vi "Log (single).vi"(8 "error in (no error)":errorcluster, 10 "Type":enum16{"Ln", "Log"}(ring), 11 "XY-data":cluster{"X-array":dbl[], "Y-array":dbl[]} {"Y-array" format="%.2p"; "X-array" format="%.2p"}) -> (0 "error out":errorcluster, 3 "XY-data out":cluster{"X-array":dbl[], "Y-array":dbl[]} {"Y-array" format="%.2p"; "X-array" format="%.2p"})   [LabVIEW 2019, in "xy_utilities.lvlib"]
doc: "Square <b>XY-data</b>'s y array.\n\nWire data to the data input to determine the polymorphic instance to use or manually select the instance."
uses:
  xy_utilities.lvlib
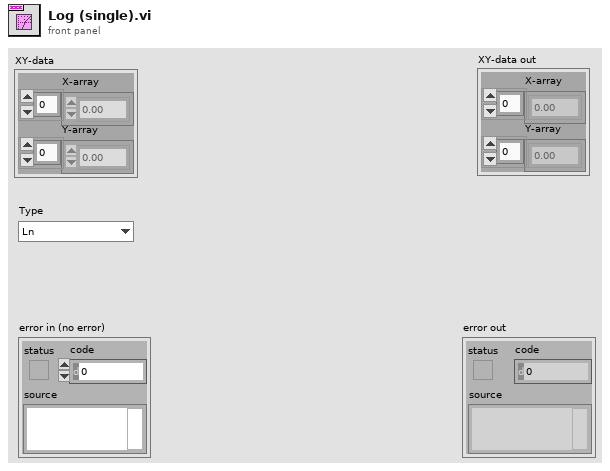
[diagram p1: front panel]
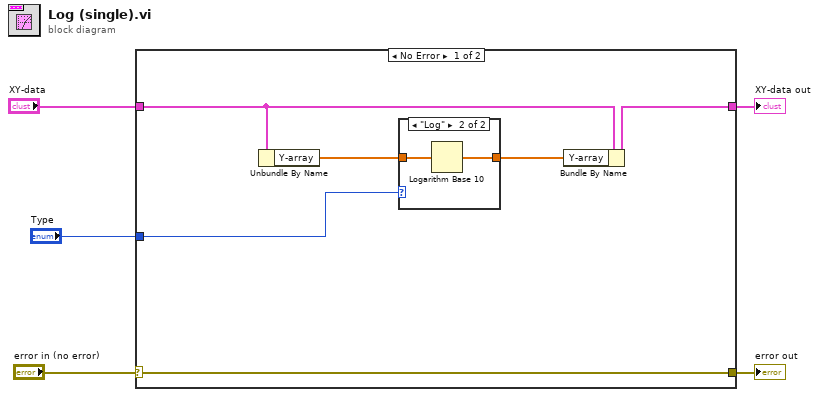
[diagram p0: block diagram]
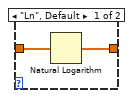
[diagram p2: hidden frame]
diagram:
  n1 = case shown="No Error" "error in (no error)" {
    selector: "error in (no error)" -> [w11 w17]
    tunnel: [w11 w17] -> w4
    tunnel: "XY-data" -> [w10 w16]
    tunnel: [w9 w16] -> w2
    tunnel: "Type" -> [w6 _]
    frame No Error {
      n2 = Unbundle By Name(w10) -> ("Y-array"=w8:dbl[])
      n3 = case shown="\"Log\"" w6 {
        tunnel: w8 -> [w13 w15]
        tunnel: [w12 w14] -> w7
        frame "Ln", Default {
          n4 = Natural Logarithm(1:w13) -> (0:w12:dbl[])
        }
        frame "Log" {
          n5 = Logarithm Base 10(1:w15) -> (0:w14:dbl[])
        }
      }
      n6 = Bundle By Name(cluster=w10, "Y-array"=w7) -> (w9:cluster{"X-array":dbl[], "Y-array":dbl[]})
    }
    frame Error {
    }
  }
  "error out" <- w4
  "XY-data out" <- w2
